vi "Keithley 2182 Ratio Calculation.vi"() -> ()   [LabVIEW 2021]
doc: "Performs a Ratio Measurement V1/V2."
uses:
  <instrlib>/Keithley 2182/Keithley 2182.lvlib
panel:
  out "Measurement":dbl
  out "Measurement Metadata":T1
  in  "V2 Reference Value (0)":dbl
  in  "V2 Enable Reference (F: Disable)":bool
  in  "V1 Reference Value (0)":dbl
  in  "V1 Enable Reference (F: Disable)":bool
  in  "Filter Type (0: Moving)":i32(ring) items=["Moving", "Repeat"]
  in  "Filter Count (10)":i32=10
  in  "Filter Window (0.01%)":dbl=0.01
  in  "Enable Digital Filter (T: Enable)":bool=TRUE
  in  "V2 Auto Range (T: Enable)":bool=TRUE
  in  "V2  Range Value (10)":dbl=10.0
  in  "Voltage Resolution (8)":i32=8
  in  "V1 Range Value (10)":dbl=10.0
  in  "V1 Auto Range (T: Enable)":bool=TRUE
  in  "Integration Rate Units (0: Line Cycles)":i32(ring) items=["Line Cycles", "Seconds"]
  in  "Integration Rate (5)":dbl=5.0
  in  "VISA resource name":refnum<visa-resource-name>
  # "(c) 2017-2018 National Instruments.  ALL RIGHTS RESERVED."
  # "General Voltage Settings"
  # "Configure V1"
  # "Ratio Calculation"
  # "Configure Filter"
  # "Configure V2"
  # "Ratio = (FiltV1 - V1Rel) / (FiltV2 - V2Rel)"
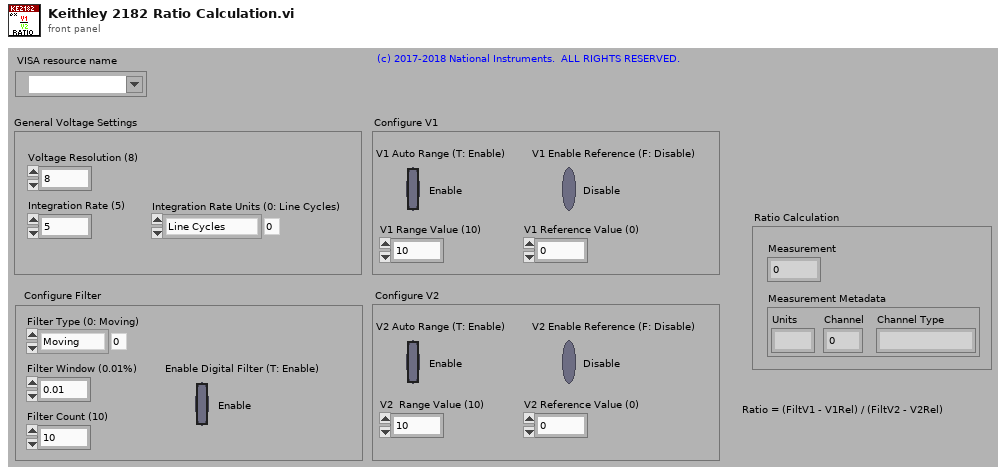
[diagram p1: front panel]
types:
  T1 = cluster{"Units":string, "Channel":i32, "Channel Type":string}
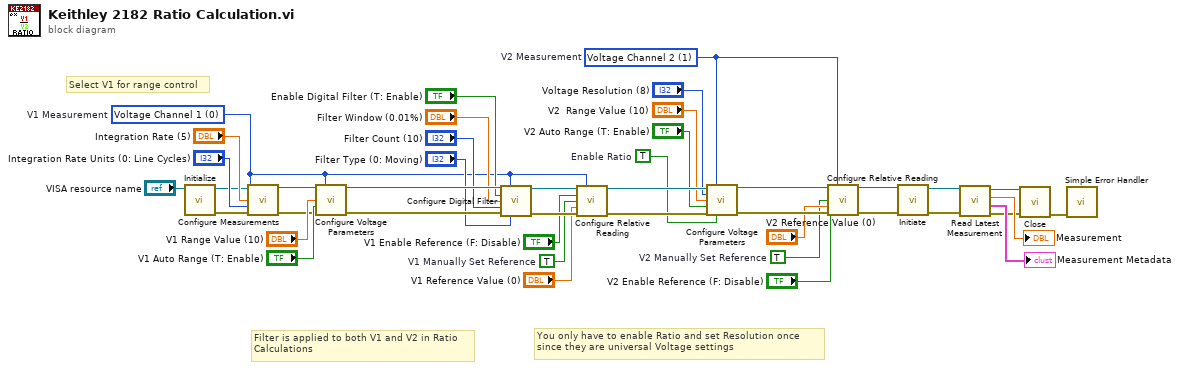
[diagram p0: block diagram]
diagram:
  w4 = 1 items=["Voltage Channel 1", "Voltage Channel 2"]  # V2 Measurement
  w18 = TRUE  # V2 Manually Set Reference
  w23 = TRUE  # V1 Manually Set Reference
  w8 = TRUE  # Enable Ratio
  w25 = 0 items=["Voltage Channel 1", "Voltage Channel 2", "Temperature Channel 1", "Temperature Channel 2"]  # V1 Measurement
  # "Select V1 for range control"
  # "Filter is applied to both V1 and V2 in Ratio\nCalculations"
  # "You only have to enable Ratio and set Resolution once\nsince they are universal Voltage settings"
  n1 = call <instrlib>:"Initialize.vi"("VISA resource name"="VISA resource name") -> ("error out"=w35:errorcluster, "VISA resource name out"=w34:refnum<visa-resource-name>)  [unwired: 9 in]
  n2 = call <instrlib>:"Configure Measurements.vi"("VISA resource name"=w34, "Measurement (0: Voltage Channel 1)"=w25, "Integration Rate (5)"="Integration Rate (5)", "Integration Rate Units (0: Line Cycles)"="Integration Rate Units (0: Line Cycles)", "error in (no error)"=w35) -> ("VISA resource name out"=w36:refnum<visa-resource-name>, "error out"=w37:errorcluster)  [unwired: 9 in]
  n3 = call <instrlib>:"Configure Voltage Parameters.vi"("VISA resource name"=w36, "Measurement (1: Voltage Channel 1)"=w25, "Range Value (12)"="V1 Range Value (10)", "Autorange (T: Enable)"="V1 Auto Range (T: Enable)", "error in (no error)"=w37) -> ("VISA resource name out"=w32:refnum<visa-resource-name>, "error out"=w33:errorcluster)  [unwired: 9 in]
  n4 = call <instrlib>:"Configure Digital Filter.vi"("VISA resource name"=w32, "Measurement (0: Voltage Channel 1)"=w25, "Enable Digital Filter (T: Enable)"="Enable Digital Filter (T: Enable)", "Filter Window (0.01%)"="Filter Window (0.01%)", "Filter Count (10)"="Filter Count (10)", "error in (no error)"=w33, "Filter Type (0: Moving)"="Filter Type (0: Moving)") -> ("VISA resource name out"=w26:refnum<visa-resource-name>, "error out"=w27:errorcluster)  [unwired: 7 in]
  n5 = call <instrlib>:"Configure Relative Reading.vi"("VISA resource name"=w26, "Measurement (0: Voltage Channel 1)"=w25, "Enable Reference (F: Disable)"="V1 Enable Reference (F: Disable)", "Manually Set Reference (F: Disable)"=w23, "Reference Value (0)"="V1 Reference Value (0)", "error in (no error)"=w27) -> ("VISA resource name out"=w9:refnum<visa-resource-name>, "error out"=w10:errorcluster)  [unwired: 8 in]
  n6 = call <instrlib>:"Configure Voltage Parameters.vi"("VISA resource name"=w9, "Measurement (1: Voltage Channel 1)"=w4, "Voltage Resolution (8)"="Voltage Resolution (8)", "Range Value (12)"="V2  Range Value (10)", "Autorange (T: Enable)"="V2 Auto Range (T: Enable)", "error in (no error)"=w10, "Enable Ratio (F: Disable)"=w8) -> ("VISA resource name out"=w20:refnum<visa-resource-name>, "error out"=w21:errorcluster)  [unwired: 7 in]
  n7 = call <instrlib>:"Configure Relative Reading.vi"("VISA resource name"=w20, "Measurement (0: Voltage Channel 1)"=w4, "Enable Reference (F: Disable)"="V2 Enable Reference (F: Disable)", "Manually Set Reference (F: Disable)"=w18, "Reference Value (0)"="V2 Reference Value (0)", "error in (no error)"=w21) -> ("VISA resource name out"=w15:refnum<visa-resource-name>, "error out"=w16:errorcluster)  [unwired: 8 in]
  n8 = call <instrlib>:"Initiate.vi"("error in (no error)"=w16, "VISA resource name"=w15) -> ("error out"=w14:errorcluster, "VISA resource name out"=w13:refnum<visa-resource-name>)  [unwired: 8 in]
  n9 = call <instrlib>:"Read Latest Measurement.vi"("error in (no error)"=w14, "VISA resource name"=w13) -> ("error out"=w2:errorcluster, "Measurement Metadata"=→"Measurement Metadata":T1, "Measurement"=→"Measurement":dbl, "VISA resource name out"=w1:refnum<visa-resource-name>)  [unwired: 6 in]
  n10 = call <instrlib>:"Close.vi"("error in (no error)"=w2, "VISA resource name"=w1) -> ("error out"=w3:errorcluster)  [unwired: 9 in]
  n11 = call <vilib>:"Simple Error Handler.vi"("error in (no error)"=w3) -> ()  [unwired: 4 in, 5 out]
